vi "Equation.vi"(1 "Distance":dbl, 2 "zAvit":dbl) -> (0 "Calculated Height":dbl)   [LabVIEW 2012]
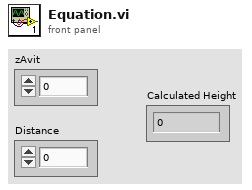
[diagram p1: front panel]
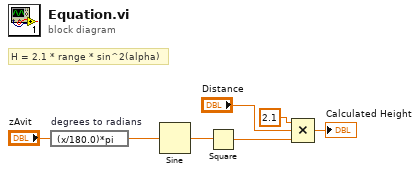
[diagram p0: block diagram]
diagram:
  # "H = 2.1 * range * sin^2(alpha)"
  n1 = expression code="(x/180.0)*pi" "degrees to radians"("zAvit") -> (w4:dbl)
  n2 = Sine(x=w4) -> (sin(x)=w3:dbl)
  n3 = Square(x=w3) -> (x^2=w2:dbl)
  n4 = Compound Arithmetic op=MULTIPLY(2.1 ("value"), "Distance", w2) -> (→"Calculated Height":dbl)
